vi "Tune Preselector.vi"(0 "VISA resource name":refnum<visa-resource-name>, 5 "Preselector (0:Auto)":i32(ring) items=["Auto", "Preset", "Set Bias"], 7 "Bias (0)":i32 min=-128 max=127, 11 "error in (no error)":errorcluster) -> (4 "VISA resource name out":refnum<visa-resource-name>, 15 "error out":errorcluster)   [LabVIEW 2020, in "Anritsu Signal Analyzer Series.lvlib"]
doc: "Sets the preselector peaking bias value."
uses:
  Anritsu Signal Analyzer Series.lvlib
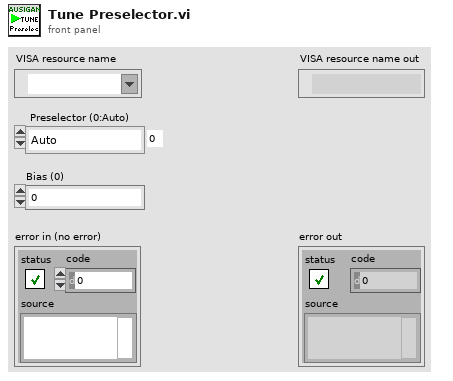
[diagram p1: front panel]
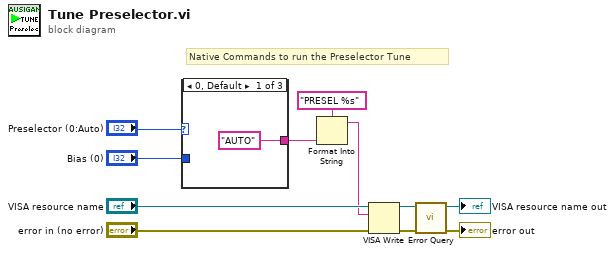
[diagram p0: block diagram]
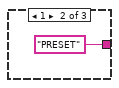
[diagram p2: hidden frame]
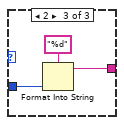
[diagram p3: hidden frame]
diagram:
  # "Native Commands to run the Preselector Tune"
  n1 = case shown="0, Default" "Preselector (0:Auto)" {
    tunnel: ["AUTO" "PRESET" w16] -> w3
    tunnel: "Bias (0)" -> [_ _ w14]
    frame 0, Default {
    }
    frame 1 {
    }
    frame 2 {
      n2 = Format Into String(format string="%d", w14) -> (resulting string=w16:string)  [unwired: 2 in, 1 out]
    }
  }
  n3 = Format Into String(format string="PRESEL %s" ("_CommandSet"), w3) -> (resulting string=w1:string)  [unwired: 2 in, 1 out]
  n4 = VISA Write(VISA resource name="VISA resource name", write buffer=w1, error in (no error)="error in (no error)") -> (VISA resource name out=w4:refnum<visa-resource-name>, error out=w5:errorcluster)  [unwired: 1 out]
  n5 = call "Error Query.vi"("error in (no error)"=w5, "VISA resource name"=w4) -> ("error out"=→"error out":errorcluster, "VISA resource name out"=→"VISA resource name out":refnum<visa-resource-name>)  [unwired: 6 in, 2 out]
